vi "Dummy Test Main.vi"() -> ()   [LabVIEW 2015]
uses:
  Exposure Process/Exposure Process.lvlib
  <vilib>/addons/PointValueMap/PointValueMap.lvlib
  ConfigHelper/ConfigHelper.lvlib
  ConfigHelper/Control_General Setup (Path).ctl
  ConfigHelper/Control_Export Setup.ctl
  System/System.lvlib
panel:
  in  "path":path=path "Z:/OneDrive - National Instruments/VM Exchange/InnoLux Fab8B 6-scans"
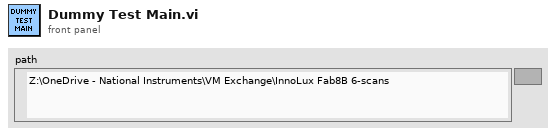
[diagram p1: front panel]
types:
  T1 = typedef "ConfigHelper.lvlib/Control_Export Setup.ctl" = cluster{"Device Name":string, "Export CSV":bool, "Export TDMS":bool, "Export RAW TDMS":bool, "Channel Names":string[]}
  T2 = typedef "ConfigHelper.lvlib/Control_General Setup (Path).ctl" = cluster{"Export Path":path, "level":dbl, "Time Gap":dbl}
  T3 = typedef "PointValueMap.lvlib/PointMap.ctl" = refnum<data-value>
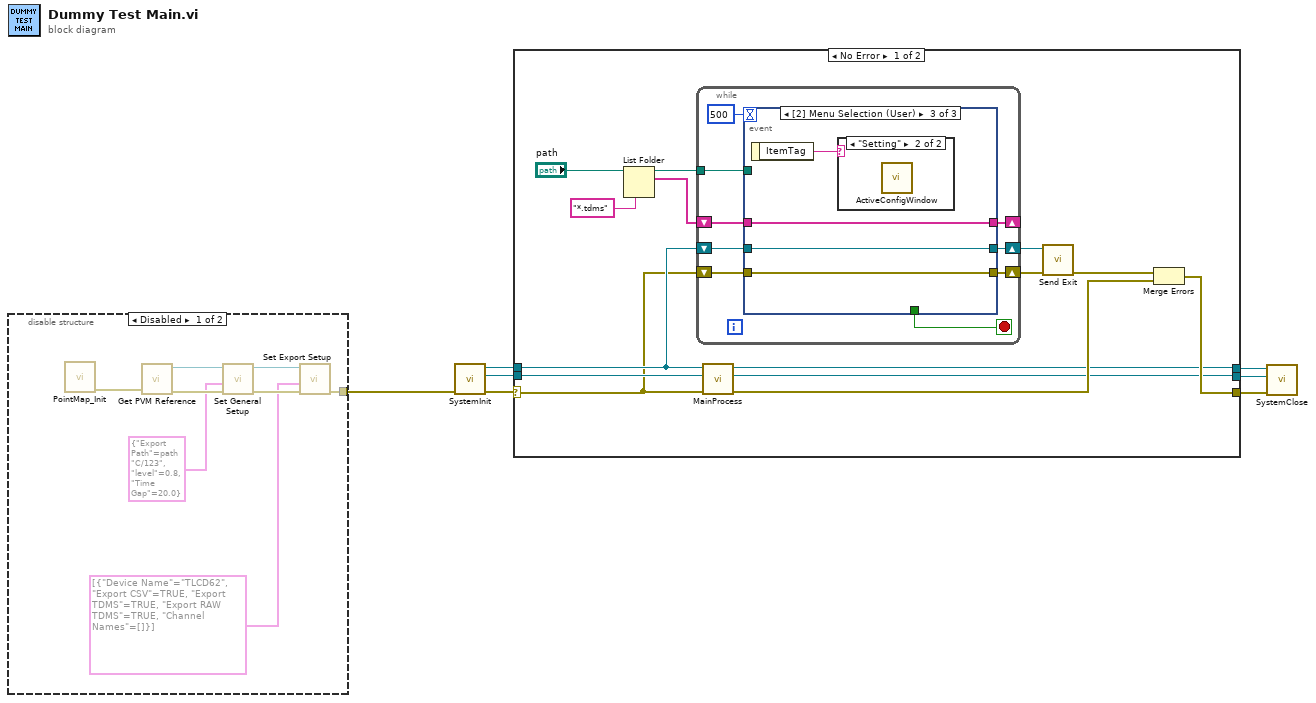
[diagram p0: block diagram]
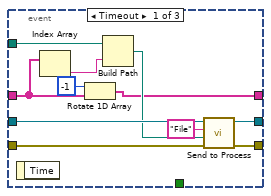
[diagram p2: hidden frame]
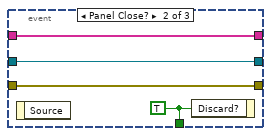
[diagram p3: hidden frame]
diagram:
  n1 = disable-structure shown="Disabled" {
    disable-tunnel: [w10 _] -> w1
    frame Disabled {
      n2 = call <vilib>:"PointMap_Init.vi"() -> ("error out"=w14:errorcluster)  [unwired: 11 in]
      n3 = call "Get PVM Reference.vi"("error in (no error)"=w14) -> ("error out"=w13:errorcluster, "Map Out"=w15:T3)  [unwired: 9 in]
      n4 = call "Set General Setup.vi"("error in (no error)"=w13, "General Setup"=T2 {"Export Path"=path "C:/123", "level"=0.8, "Time Gap"=20.0}, "Map"=w15) -> ("error out"=w11:errorcluster, "Map Out"=w12:T3)  [unwired: 7 in]
      n5 = call "Set Export Setup.vi"("error in (no error)"=w11, "Export Setup"=T1[] [{"Device Name"="TLCD62", "Export CSV"=TRUE, "Export TDMS"=TRUE, "Export RAW TDMS"=TRUE, "Channel Names"=[]}], "Map"=w12) -> ("error out"=w10:errorcluster)  [unwired: 7 in, 1 out]
    }
    frame Enabled {
    }
  }
  n6 = call "SystemInit.vi"("error in (no error)"=w1) -> ("error out"=w5:errorcluster, "Pound"=w6:refnum<class "Pound.lvclass">, "Qbus out"=w7:refnum<class "Qbus.lvclass">)  [unwired: 8 in]
  n7 = case shown="No Error" w5 {
    selector: w5 -> [w19 w58]
    tunnel: w7 -> [w21 w60]
    tunnel: w6 -> [w20 w59]
    tunnel: [w17 w60] -> w4
    tunnel: [w16 w59] -> w3
    tunnel: [w23 w58] -> w2
    frame No Error {
      n8 = List Folder(path="path", pattern="*.tdms") -> (path out=w27:path, filenames=w22:string[])  [unwired: 2 in, 2 out]
      n9 = while {
        tunnel: w27 -> [w38]
        shift-right: [w35] -> w26
        shift-left: w21 -> [w37]
        shift-right: [w34] -> w25
        shift-left: w19 -> [w36]
        shift-right: [w32] -> _
        shift-left: w22 -> [w33]
        stop <- w30 stop-if-true
        n10 = event shown="[2] Menu Selection (User)" {
          selector: _ -> [_ _ _]
          dyn-events: _ -> [_ _ _]
          timeout: 500 -> [_ _ _]
          tunnel: w38 -> [w49 _ _]
          tunnel: w37 -> [w48 w52 w56]
          tunnel: w36 -> [w47 w53 w55]
          tunnel: [w44 w52 w56] -> w35
          tunnel: [w43 w53 w55] -> w34
          tunnel: w33 -> [w41 w51 w57]
          tunnel: [w40 w51 w57] -> w32
          tunnel: [_ w50 _] -> w30
          event Timeout {
            n11 = event-data() -> ()  [unwired: 1 in, 1 out]
            n12 = Index Array(array=w41) -> (element=w42:string)  [unwired: 1 in]
            n13 = Rotate 1D Array(1:w41, 2:-1 ("n")) -> (0:w40:string[])
            n14 = Build Path(base path=w49, name or relative path=w42) -> (appended path=w46:path)
            n15 = call "Send to Process.vi"("error in (no error)"=w47, "message value"=w46, "message name"="File", "qbus in"=w48) -> ("error out"=w43:errorcluster, "qbus out"=w44:refnum<class "Qbus.lvclass">)  [unwired: 6 in]
          }
          event Panel Close? {
            w50 = TRUE ("Discard?")
            n16 = event-data() -> ()  [unwired: 1 in, 1 out]
            n17 = event-data("Discard?"=w50) -> ()  [unwired: 1 in, 1 out]
          }
          event Menu Selection (User) {
            n18 = event-data() -> ("ItemTag"=w54:string)  [unwired: 1 in]
            n19 = case shown="\"Setting\"" w54 {
              frame Default {
              }
              frame "Setting" {
                n20 = call "ActiveConfigWindow.vi"() -> ()  [unwired: 12 in]
              }
            }
          }
        }
      }
      n21 = call "MainProcess.vi"("error in (no error)"=w19, "pound in"=w20, "qbus in"=w21) -> ("error out"=w18:errorcluster, "Pound"=w16:refnum<class "Pound.lvclass">, "Qbus out"=w17:refnum<class "Qbus.lvclass">)  [unwired: 6 in]
      n22 = call "Send Exit.vi"("error in (no error)"=w25, "qbus in"=w26) -> ("error out"=w24:errorcluster)  [unwired: 8 in, 1 out]
      n23 = Merge Errors(w24, w18) -> (w23:errorcluster)
    }
    frame Error {
    }
  }
  n24 = call "SystemClose.vi"("error in (no error)"=w2, "Pound"=w3, "Qbus"=w4) -> ()  [unwired: 8 in, 1 out]
